vi "TreeNode Destroy.vi"(8 "error in (no error)":errorcluster, 11 "TreeNode DVR in":refnum<data-value>) -> (0 "error out":errorcluster)   [LabVIEW 2015, in "MDSplus.lvlib"]
uses:
  <vilib>/MDSplus/Library/MDSplus.lvlib
  <vilib>/MDSplus/Classes/Data_Class/TreeNode_Class/TreeNode.lvclass
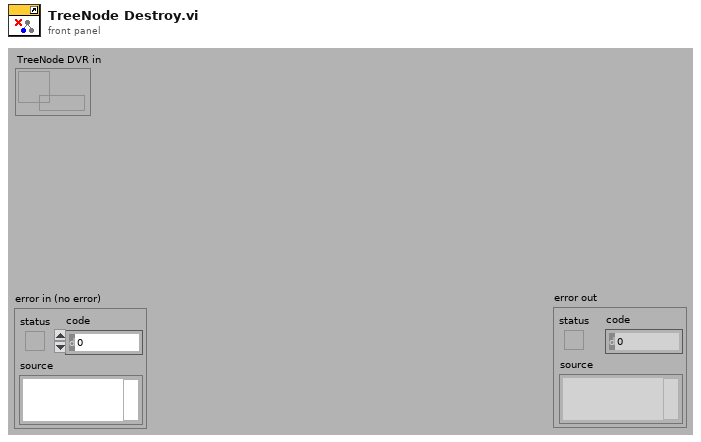
[diagram p1: front panel]
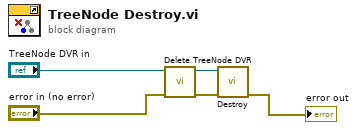
[diagram p0: block diagram]
diagram:
  n1 = call <vilib>:"Delete TreeNode DVR.vi"("error in (no error)"="error in (no error)", "TreeNode DVR in"="TreeNode DVR in") -> ("error out"=w4:errorcluster, "TreeNode out"=w5:refnum<class "TreeNode.lvclass">)  [unwired: 8 in]
  n2 = call-dynamic "Destroy.vi"("error in (no error)"=w4, "TreeNode in"=w5) -> ("error out"=→"error out":errorcluster)  [unwired: 9 in]
